vi "Test Stack.vi"() -> ()   [LabVIEW 2012, in "Stack.lvlib"]
doc: "VI is used to demonstrate the usage of stack."
uses:
  Stack.lvlib
  Stack.lvclass
panel:
  out "Element":dbl
  out "Stack":dbl[](array[numeric])
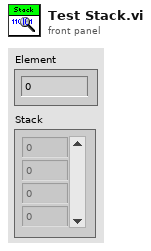
[diagram p1: front panel]
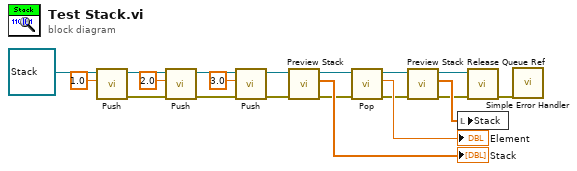
[diagram p0: block diagram]
diagram:
  n1 = call "Push.vi"("Element"=1.0, "Stack in"=refnum<class "Stack.lvclass"> refnum ("Stack.lvlib:Stack.lvclass")) -> ("error out"=w16:errorcluster, "Stack out"=w17:refnum<class "Stack.lvclass">)  [unwired: 8 in]
  n2 = call "Push.vi"("error in (no error)"=w16, "Element"=2.0, "Stack in"=w17) -> ("error out"=w13:errorcluster, "Stack out"=w14:refnum<class "Stack.lvclass">)  [unwired: 7 in]
  n3 = call "Push.vi"("error in (no error)"=w13, "Element"=3.0, "Stack in"=w14) -> ("error out"=w11:errorcluster, "Stack out"=w12:refnum<class "Stack.lvclass">)  [unwired: 7 in]
  n4 = call "Preview Stack.vi"("error in (no error)"=w11, "Stack in"=w12) -> ("error out"=w8:errorcluster, "Stack"=→"Stack":dbl[], "Stack out"=w9:refnum<class "Stack.lvclass">)  [unwired: 7 in]
  n5 = call "Pop.vi"("error in (no error)"=w8, "Stack in"=w9) -> ("error out"=w6:errorcluster, "Element"=→"Element":dbl, "Stack out"=w5:refnum<class "Stack.lvclass">)  [unwired: 7 in]
  n6 = call "Preview Stack.vi"("error in (no error)"=w6, "Stack in"=w5) -> ("error out"=w2:errorcluster, "Stack"=w4:dbl[], "Stack out"=w3:refnum<class "Stack.lvclass">)  [unwired: 7 in]
  n7 = local write "Stack"(w4) -> ()
  n8 = call "Release Queue Ref.vi"("error in (no error)"=w2, "Stack in"=w3) -> ("error out"=w1:errorcluster)  [unwired: 9 in]
  n9 = call <vilib>:"Simple Error Handler.vi"("error in (no error)"=w1) -> ()  [unwired: 4 in, 5 out]
